vi "Bulk Create.vi"(4 "TypeMap in":refnum<class "TypeMap.lvclass">, 6 "commandTimeout":i32=-1, 8 "error in (no error)":errorcluster, 10 "object in":refnum<class>[](array[class]), 11 "SqlMapper in":refnum<class "SqlMapper.lvclass">) -> (0 "error out":errorcluster, 1 "id":i32[](array[numeric]), 2 "object out":refnum<class>[](array[class]), 3 "SqlMapper out":refnum<class "SqlMapper.lvclass">)   [LabVIEW 2020, in "ORM_API.lvlib"]
doc: "NSERT a single entities."
uses:
  ORM_API.lvlib
  <vilib>/Viviota/shared/ORM.lvlibp/ORM/TypeMap/TypeMap.lvclass
  <vilib>/Viviota/shared/ORM.lvlibp/ORM/SqlMapper/SqlMapper.lvclass
  <userlib>/_OpenG.lib/lvdata/lvdata.llb/LVOOP Is Default Value__ogtk.vi
  <vilib>/Viviota/shared/ORM.lvlibp/ORM/TypeMap/Read TypeMap.vi
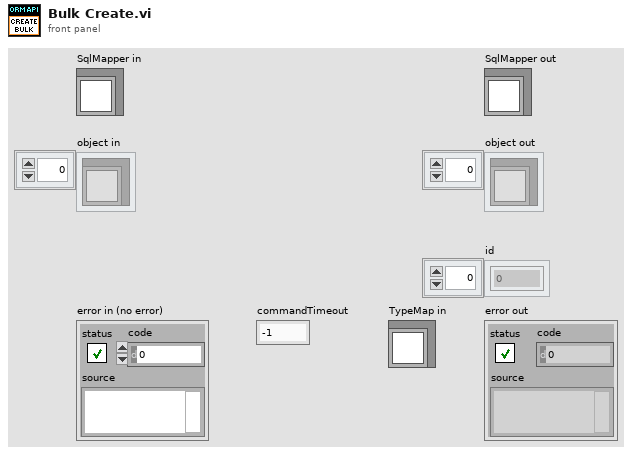
[diagram p1: front panel]
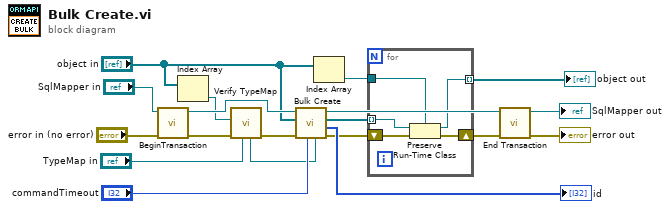
[diagram p0: block diagram]
diagram:
  n1 = call-dynamic "BeginTransaction.vi"("error in (no error)"="error in (no error)", "SqlMapper in"="SqlMapper in") -> ("error out"=w14:errorcluster, "SqlMapper out"=w16:refnum<class "SqlMapper.lvclass">)  [unwired: 8 in]
  n2 = Index Array(array="object in") -> (element=w5:refnum<class>)  [unwired: 1 in]
  n3 = call "Verify TypeMap.vi"("TypeMap in"="TypeMap in", "error in (no error)"=w14, "Type in"=w5) -> ("error out"=w12:errorcluster, "TypeMap out"=w10:refnum<class "TypeMap.lvclass">)  [unwired: 6 in, 1 out]
  n4 = call-dynamic "Bulk Create.vi"("TypeMap in"=w10, "commandTimeout"="commandTimeout", "error in (no error)"=w12, "object in"="object in", "SqlMapper in"=w16) -> ("error out"=w4:errorcluster, "id"=→"id":i32[], "object out"=w3:refnum<class>[], "SqlMapper out"=w18:refnum<class "SqlMapper.lvclass">)  [unwired: 3 in]
  n5 = Index Array(array="object in") -> (element=w2:refnum<class>)  [unwired: 1 in]
  n6 = for {
    tunnel: [w23] -> w6 mode=indexing
    tunnel: w2 -> [w22]
    tunnel: w3 -> [w20] mode=indexing
    shift-right: [w24] -> w7
    shift-left: w4 -> [w21]
    n7 = Preserve Run-Time Class(object in=w20, error in=w21, 2:w22) -> (object out=w23:refnum<class>, error out=w24:errorcluster)
  }
  "object out" <- w6
  n8 = call <vilib>:"End Transaction.vi"("error in (no error)"=w7, "SqlMapper in"=w18) -> ("error out"=→"error out":errorcluster, "SqlMapper out"=→"SqlMapper out":refnum<class "SqlMapper.lvclass">)  [unwired: 8 in]
